vi "ConfigureProximitySensor.vi"(8 "error in (no error)":errorcluster, 9 "ProximitySensorMeasurementRate":T1, 10 "ProximitySensorResolution":T2, 11 "ColorSensorDevRef":T3={"I2CDevRef"={"DevStatus"={"status"=FALSE, "code"=0, "source"=""}, "Device Address"=0, "Handle"=0, "I2C Bus"=enum."Invalid"}} {"I2CDevRef"."Device Address" format="%.0x"}) -> (0 "error out":errorcluster, 3 "ColorSensorDevRef out":T3={"I2CDevRef"={"DevStatus"={"status"=FALSE, "code"=0, "source"=""}, "Device Address"=0, "Handle"=0, "I2C Bus"=enum."Invalid"}} {"I2CDevRef"."Device Address" format="%.0x"})   [LabVIEW 2018, in "ColorSensor.lvlib"]
uses:
  ColorSensor.lvlib
  TypeDef/ColorSensorDevRef.ctl
  <vilib>/Rock Robotics/WPI/I2C/WPI_I2CDevRef.ctl
  <vilib>/Rock Robotics/SystemInterfaces/i2clib/i2c_bus.ctl
  TypeDef/ProximitySensorResolution.ctl
  TypeDef/ProximitySensorMeasurementRate.ctl
  Private/Registers.ctl
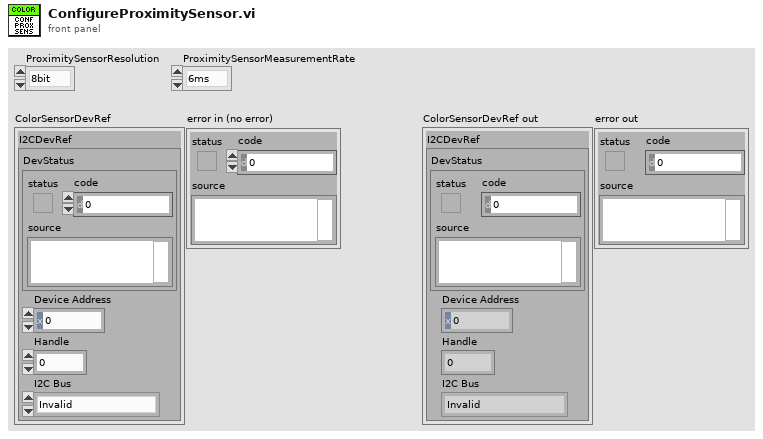
[diagram p1: front panel]
types:
  T1 = typedef "ColorSensor.lvlib/ProximitySensorMeasurementRate.ctl" = enum16{"6ms", "12ms", "25ms", "50ms", "100ms", "200ms", "400ms"}
  T2 = typedef "ColorSensor.lvlib/ProximitySensorResolution.ctl" = enum8{"8bit", "9bit", "10bit", "11bit"}
  T3 = typedef "ColorSensor.lvlib/ColorSensorDevRef.ctl" = cluster{"I2CDevRef":T4}
  T4 = typedef "WPI_I2CDevRef.ctl" = cluster{"DevStatus":errorcluster, "Device Address":u8, "Handle":i32, "I2C Bus":T5}
  T5 = typedef "i2c_bus.ctl" = enum16{"I2C On-Board", "I2C MXP", "Invalid"}
  T6 = typedef "ColorSensor.lvlib/Registers.ctl" = enum16{"MainCtrl", "ProximitSensorLED", "ProximitySensorPulse", "ProximitySensorRate", "LightSensorMeasurementRate", "LightSensorGainRegister", "PartIDRegister", "MainStatus", "ProximityData", "ProximityData1", "InfraredData", "InfraredData1", "InfraredData2", "GreenData", "GreenData1", "GreenData2", "BlueData", "BlueData1", "BlueData2", "RedData", "RedData1", "RedData2"}
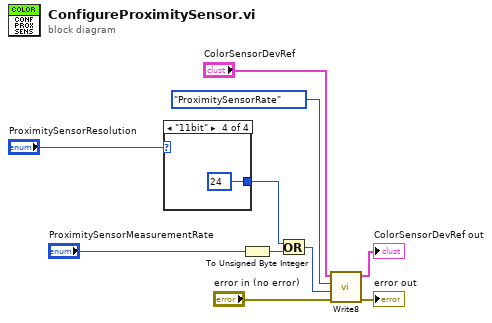
[diagram p0: block diagram]
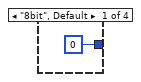
[diagram p2: hidden frame]
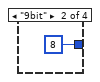
[diagram p3: hidden frame]
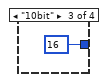
[diagram p4: hidden frame]
diagram:
  n1 = case shown="\"11bit\"" "ProximitySensorResolution" {
    tunnel: [u8 0 ("Data") u8 8 ("Data") u8 16 ("Data") u8 24 ("Data")] -> w2
    frame "8bit", Default {
    }
    frame "9bit" {
    }
    frame "10bit" {
    }
    frame "11bit" {
    }
  }
  n2 = To Unsigned Byte Integer(number="ProximitySensorMeasurementRate") -> (unsigned 8bit integer=w3:u8)
  n3 = Or(x=w2, y=w3) -> (x .or. y?=w1:u8)
  n4 = call "Write8.vi"("error in (no error)"="error in (no error)", "Data"=w1, "Registers"=Registers."ProximitySensorRate", "ColorSensorDevRef"="ColorSensorDevRef") -> ("error out"=→"error out":errorcluster, "ColorSensorDevRef out"=→"ColorSensorDevRef out":T3)  [unwired: 6 in]
